vi "add_sequence.vi"(8 "error in":errorcluster, 11 "sequence in":dbl[](array[numeric])) -> (0 "error out":errorcluster, 3 "sequence out":dbl[](array[numeric]))   [LabVIEW 2024]
uses:
  <vilib>/numeric/Random Number (Range) U64.vi
  <vilib>/numeric/sub_Random U32.vi
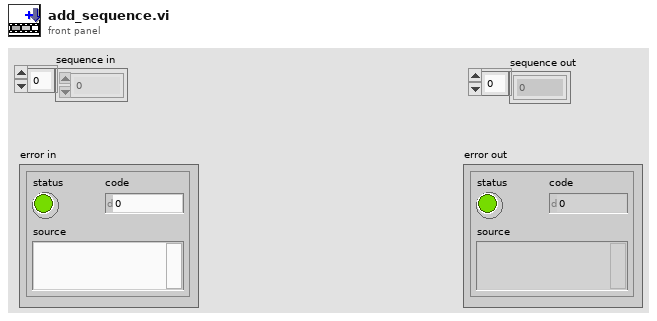
[diagram p1: front panel]
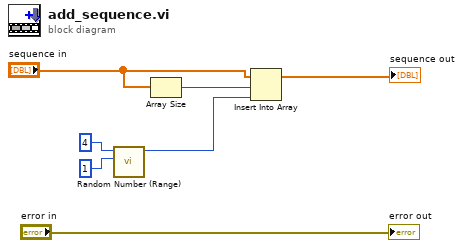
[diagram p0: block diagram]
diagram:
  n1 = call-poly <vilib>:"Random Number (Range).vi"("lower bound (0)"=u64 1, "upper bound (100)"=u64 4) -> ("number"=w2:u64)  [unwired: 9 in]
  n2 = Array Size(array="sequence in") -> (size(s)=w7:i32)
  n3 = Insert Into Array(array="sequence in", index=w7, new element=w2) -> (→"sequence out":dbl[])
  "error out" <- "error in"
